vi "Render.vi"(8 "error in":errorcluster, 11 "class data in":refnum<class "Game.lvclass">) -> (0 "error out":errorcluster, 2 "quit out":bool, 3 "class data out":refnum<class "Game.lvclass">)   [LabVIEW 2010, in "Labricks.lvlib" / "Game.lvclass"]
uses:
  Game.lvclass
  Brick_class/Brick.lvclass
  Game.lvclass/Game.ctl
  BoundingBox_class/BoundingBox.lvclass
  Paddle_class/Paddle.lvclass
  RenderBase/SceneRoot_class/SceneRoot.lvclass
  Text_class/properties/Text/SetText.vi
  Text_class/Text.lvclass
  RenderBase/Sprite_class/Sprite.lvclass
  Ball_class/Ball.lvclass
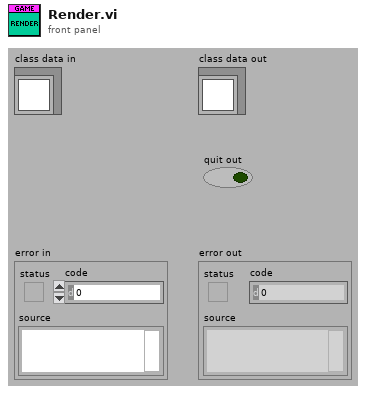
[diagram p1: front panel]
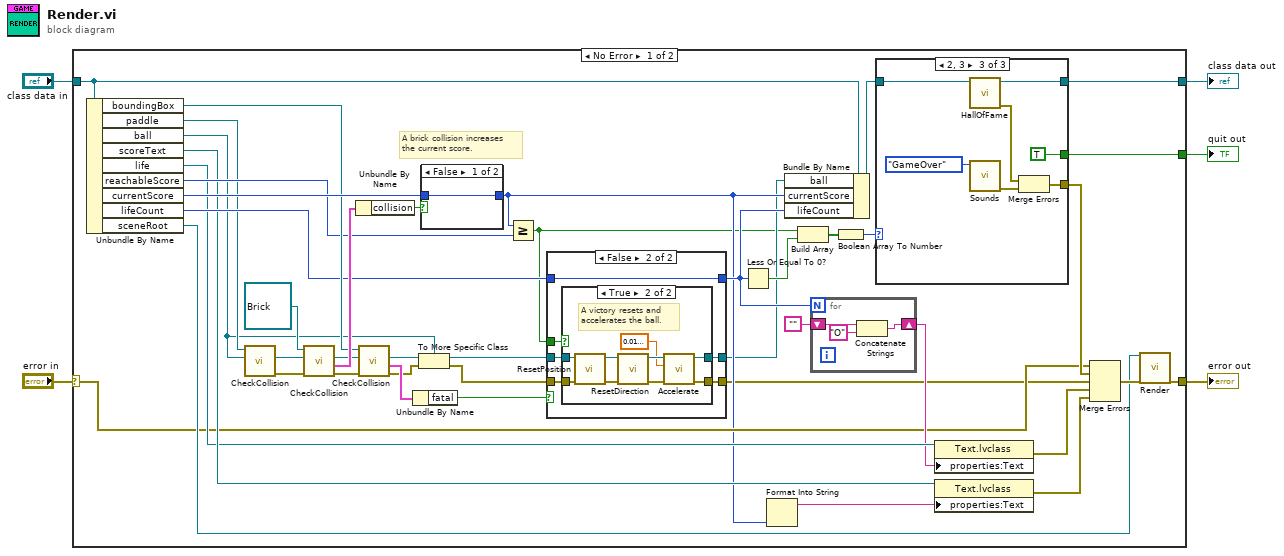
[diagram p0: block diagram]
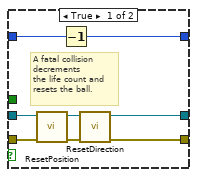
[diagram p2: hidden frame]
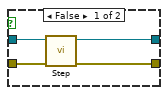
[diagram p3: hidden frame]
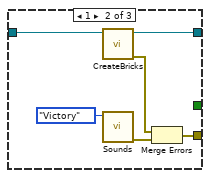
[diagram p5: hidden frame]
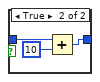
[diagram p6: hidden frame]
diagram:
  n1 = case shown="No Error" "error in" {
    selector: "error in" -> [w16 w98]
    tunnel: "class data in" -> [w20 w97]
    tunnel: [w18 w97] -> w2
    tunnel: [w39 w98] -> w3
    tunnel: [w17 _] -> w1
    frame No Error {
      # "A brick collision increases\nthe current score."
      n2 = Unbundle By Name(w20) -> ("boundingBox"=w43:refnum<class "BoundingBox.lvclass">, "paddle"=w36:refnum<class "Paddle.lvclass">, "ball"=w7:refnum<class "Ball.lvclass">, "scoreText"=w40:refnum<class "Text.lvclass">, "life"=w25:refnum<class "Text.lvclass">, "reachableScore"=w42:i32, "currentScore"=w44:i32, "lifeCount"=w41:i32, "sceneRoot"=w35:refnum<class "SceneRoot.lvclass">)
      n3 = call-dynamic "CheckCollision.vi"("sprite in"=w7, "class data in"=w36) -> ("error out"=w32:errorcluster, "sprite out"=w30:refnum<class "Sprite.lvclass">)  [unwired: 6 in, 2 out]
      n4 = call-dynamic "CheckCollision.vi"("error in"=w32, "sprite in"=w30, "class data in"=refnum<class "Brick.lvclass"> refnum ("brick in")) -> ("error out"=w31:errorcluster, "collisionInfo out"=w45:cluster{"collision":bool, "fatal":bool}, "sprite out"=w28:refnum<class "Sprite.lvclass">)  [unwired: 5 in, 1 out]
      n5 = Unbundle By Name(w45) -> ("collision"=w48:bool)
      n6 = call-dynamic "CheckCollision.vi"("error in"=w31, "sprite in"=w28, "class data in"=w43) -> ("error out"=w33:errorcluster, "collisionInfo out"=w47:cluster{"collision":bool, "fatal":bool}, "sprite out"=w34:refnum<class "Sprite.lvclass">)  [unwired: 5 in, 1 out]
      n7 = Unbundle By Name(w47) -> ("fatal"=w15:bool)
      n8 = To More Specific Class(target class=w7, reference=w34, error in=w33) -> (specific class reference=w11:refnum<class "Ball.lvclass">, error out=w10:errorcluster)
      n9 = case shown="False" w48 {
        tunnel: [w93 w94] -> w12
        tunnel: w44 -> [w93 w96]
        frame False {
        }
        frame True {
          n10 = Add(x=w96, y=10) -> (x+y=w94:i32)
        }
      }
      n11 = Greater Or Equal?(x=w12, y=w42) -> (x >= y?=w6:bool)
      n12 = case shown="False" w15 {
        tunnel: w41 -> [w56 w58]
        tunnel: [w55 w58] -> w14
        tunnel: w11 -> [w52 w62]
        tunnel: w10 -> [w51 w61]
        tunnel: [w50 w60] -> w9
        tunnel: [w49 w59] -> w8
        tunnel: w6 -> [_ w57]
        frame True {
          # "A fatal collision\ndecrements\nthe life count and\nresets the ball."
          n13 = call "ResetPosition.vi"("error in"=w51, "class data in"=w52) -> ("error out"=w54:errorcluster, "class data out"=w53:refnum<class "Ball.lvclass">)  [unwired: 8 in]
          n14 = Decrement(x=w56) -> (x-1=w55:i32)
          n15 = call "ResetDirection.vi"("error in"=w54, "class data in"=w53) -> ("error out"=w49:errorcluster, "class data out"=w50:refnum<class "Ball.lvclass">)  [unwired: 8 in]
        }
        frame False {
          n16 = case shown="True" w57 {
            tunnel: w62 -> [w64 w73]
            tunnel: w61 -> [w66 w72]
            tunnel: [w63 w69] -> w60
            tunnel: [w65 w68] -> w59
            frame False {
              n17 = call "Step.vi"("error in"=w66, "class data in"=w64) -> ("error out"=w65:errorcluster, "class data out"=w63:refnum<class "Ball.lvclass">)  [unwired: 8 in]
            }
            frame True {
              # "A victory resets and\naccelerates the ball."
              n18 = call "ResetPosition.vi"("error in"=w72, "class data in"=w73) -> ("error out"=w75:errorcluster, "class data out"=w74:refnum<class "Ball.lvclass">)  [unwired: 8 in]
              n19 = call "ResetDirection.vi"("error in"=w75, "class data in"=w74) -> ("error out"=w70:errorcluster, "class data out"=w71:refnum<class "Ball.lvclass">)  [unwired: 8 in]
              n20 = call "Accelerate.vi"("error in (no error)"=w70, "increment"=sgl 0.02, "class data in"=w71) -> ("error out"=w68:errorcluster, "class data out"=w69:refnum<class "Ball.lvclass">)  [unwired: 7 in]
            }
          }
        }
      }
      n21 = Less Or Equal To 0?(x=w14) -> (x <= 0?=w13:bool)
      n22 = Format Into String(w12) -> (resulting string=w46:string)  [unwired: 3 in, 1 out]
      n23 = Bundle By Name(cluster=w20, "ball"=w9, "currentScore"=w12, "lifeCount"=w14) -> (w19:refnum<class "Game.lvclass">)
      n24 = Build Array(w6, w13) -> (w37:bool[])
      n25 = for {
        N: w14 -> [_]
        shift-right: [w91] -> w24
        shift-left: "" -> [w92]
        n26 = Concatenate Strings(w92, "O" ("string")) -> (w91:string)
      }
      n27 = Boolean Array To Number(Boolean array=w37) -> (number=w22:u32)
      n28 = case shown="2, 3" w22 {
        tunnel: w19 -> [w76 w82 w84]
        tunnel: [w76 w81 w83] -> w18
        tunnel: [_ w78 w87] -> w21
        tunnel: [_ _ TRUE] -> w17
        frame 0, Default {
        }
        frame 1 {
          n29 = call "CreateBricks.vi"("class data in"=w82) -> ("error out"=w80:errorcluster, "class data out"=w81:refnum<class "Game.lvclass">)  [unwired: 9 in]
          n30 = call "Sounds.vi"("choice in"=enum16{"Victory", "GameOver"}."Victory") -> ("error out"=w77:errorcluster)  [unwired: 10 in]
          n31 = Merge Errors(w80, w77) -> (w78:errorcluster)
        }
        frame 2, 3 {
          n32 = call "HallOfFame.vi"("class data in"=w84) -> ("error out"=w88:errorcluster, "class data out"=w83:refnum<class "Game.lvclass">)  [unwired: 9 in]
          n33 = call "Sounds.vi"("choice in"=enum16{"Victory", "GameOver"}."GameOver") -> ("error out"=w86:errorcluster)  [unwired: 10 in]
          n34 = Merge Errors(w88, w86) -> (w87:errorcluster)
        }
      }
      n35 = property class="Text.lvclass"(reference=w25, "properties:Text"=w24) -> (error out=w26:errorcluster)  [unwired: 1 in, 1 out]
      n36 = property class="Text.lvclass"(reference=w40, "properties:Text"=w46) -> (error out=w27:errorcluster)  [unwired: 1 in, 1 out]
      n37 = Merge Errors(w16, w21, w8, w26, w27) -> (w38:errorcluster)
      n38 = call-dynamic "Render.vi"("class data in"=w35, "error in (no error)"=w38) -> ("error out"=w39:errorcluster)  [unwired: 16 in, 1 out]
    }
    frame Error {
    }
  }
  "class data out" <- w2
  "error out" <- w3
  "quit out" <- w1
